vi "自我介绍.vi"(8 "error in (no error)":errorcluster caption="错误输入（无错误）", 11 "鸭子 输入":refnum<class "鸭子.lvclass">) -> (0 "error out":errorcluster caption="错误输出", 3 "鸭子 输出":refnum<class "鸭子.lvclass">)   [LabVIEW 2018, in "鸭子库.lvlib" / "鸭子.lvclass"]
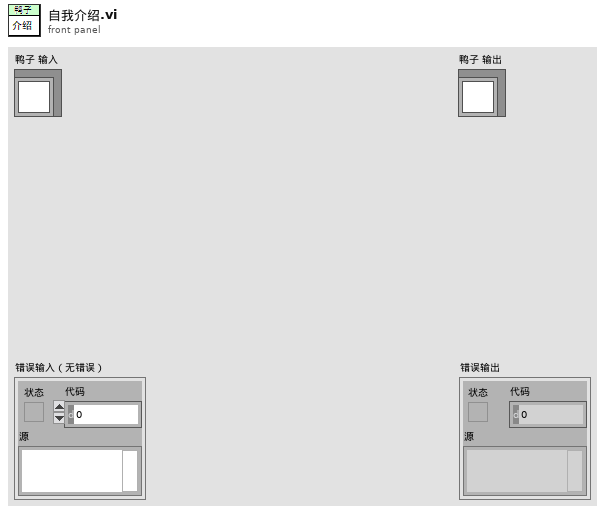
[diagram p1: front panel]
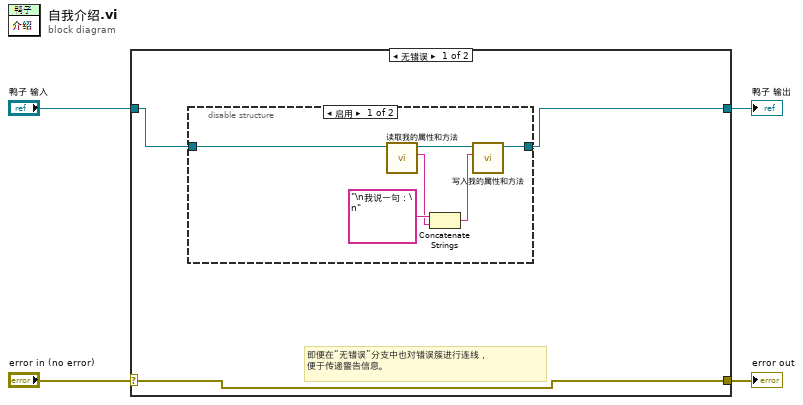
[diagram p0: block diagram]
diagram:
  n1 = case shown="无错误" "error in (no error)" {
    selector: "error in (no error)" -> [w7 w16]
    tunnel: [w7 w16] -> w3
    tunnel: [w6 w15] -> w1
    tunnel: "鸭子 输入" -> [w5 w15]
    frame No Error {
      # "即便在“无错误”分支中也对错误簇进行连线，\n便于传递警告信息。"
      n2 = disable-structure shown="启用" {
        disable-tunnel: [w13 w14] -> w6
        disable-tunnel: w5 -> [w8 w14]
        frame Enabled {
          n3 = call "读取我的属性和方法.vi"("鸭子输入"=w8) -> ("我的属性和方法"=w10:string, "鸭子输出"=w9:refnum<class "鸭子.lvclass">)  [unwired: 8 in, 1 out]
          n4 = Concatenate Strings("\n我说一句：\n" ("字符串"), w10) -> (w12:string)
          n5 = call "写入我的属性和方法.vi"("我的属性和方法"=w12, "鸭子输入"=w9) -> ("鸭子输出"=w13:refnum<class "鸭子.lvclass">)  [unwired: 8 in, 1 out]
        }
        frame Disabled {
        }
      }
    }
    frame Error {
    }
  }
  "error out" <- w3
  "鸭子 输出" <- w1
